vi "LV_beta.vi"() -> ()   [LabVIEW 2021]
uses:
  <vilib>/Analysis/NI_AALBase.lvlib
panel:
  out "Unscrambled":string
  out "Scrambled":string
  in  "Path 2":path
  out "Waveform Graph":dbl[](graph)
  out "length":i32
  in  "Path":path
  out "Display":string
  in  "CALC UI":T1
  in  "stop":bool
  out "Waveform Chart":dbl[](graph)
  out "String":string
  out "number (0 to 1)":dbl
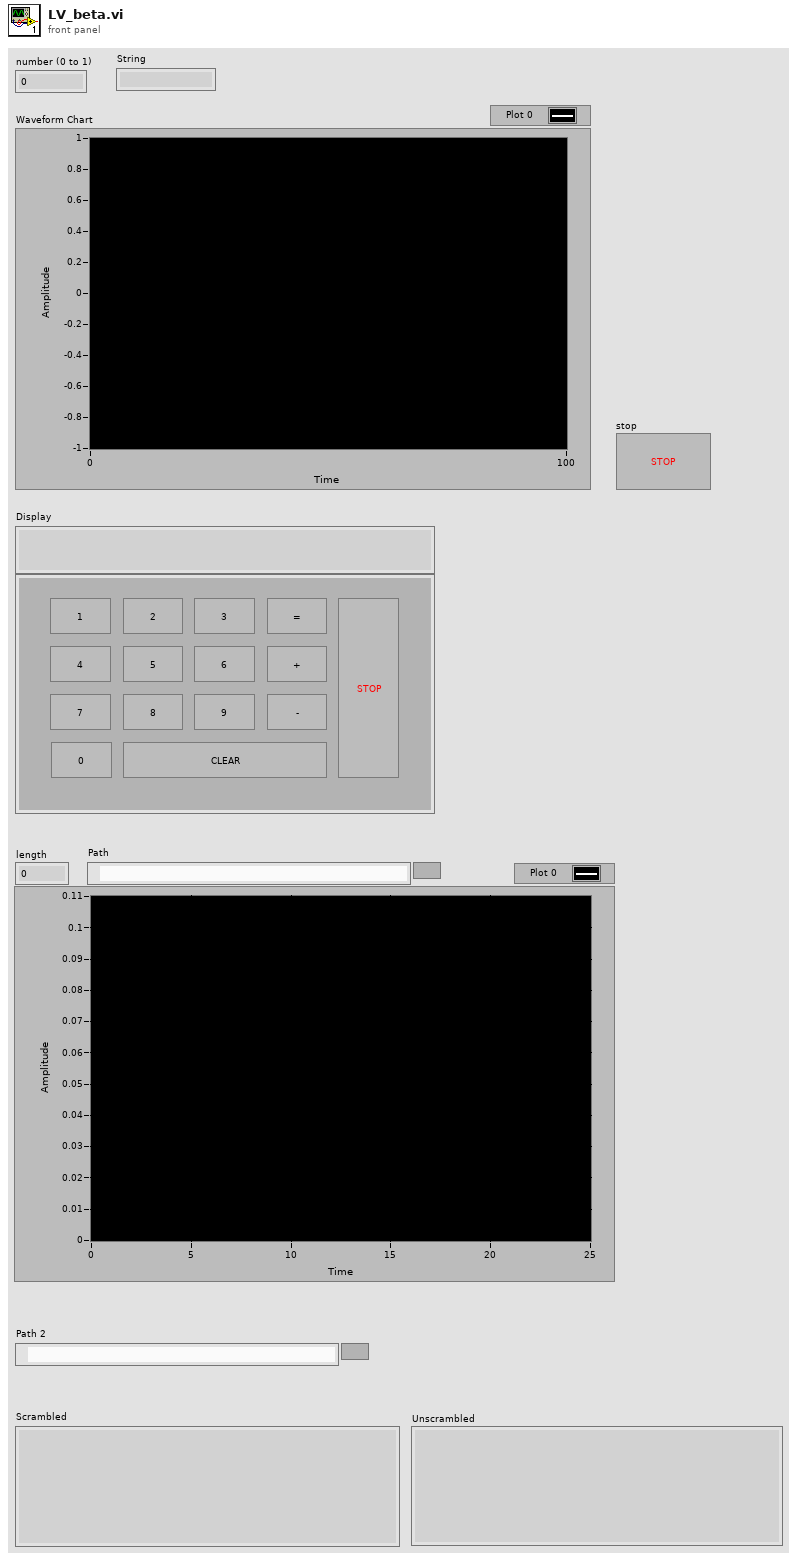
[diagram p1: front panel]
types:
  T1 = cluster{"1":bool, "2":bool, "3":bool, "Result":bool, "4":bool, "5":bool, "6":bool, "Add":bool, "7":bool, "8":bool, "9":bool, "Subtract":bool, "0":bool, "CLEAR":bool, "stop":bool}
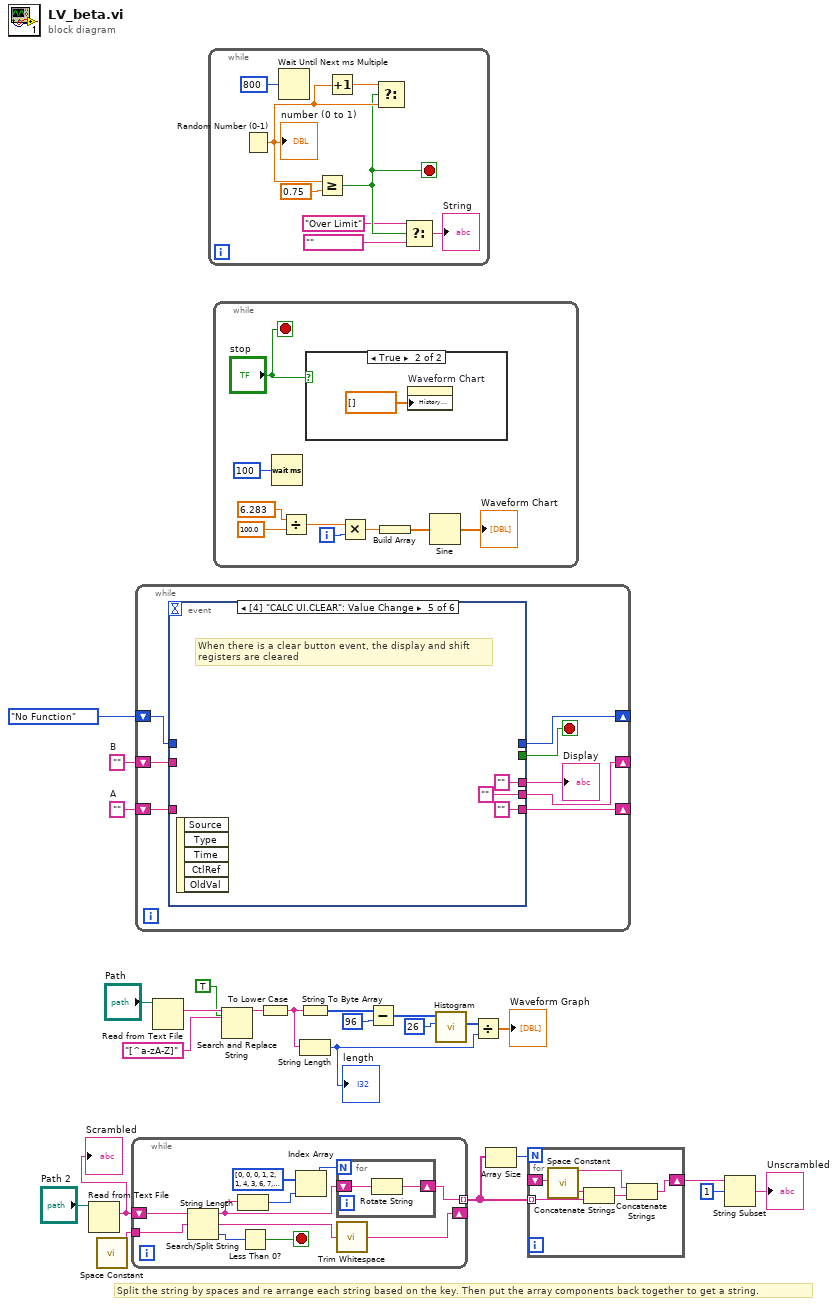
[diagram p0: block diagram]
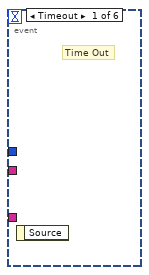
[diagram p2: hidden frame]
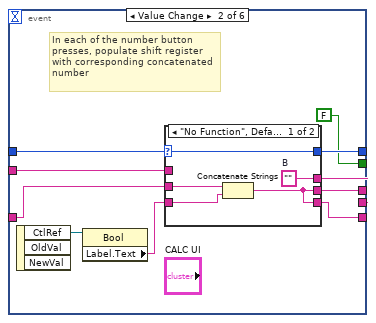
[diagram p3: hidden frame]
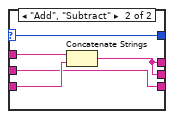
[diagram p4: hidden frame]
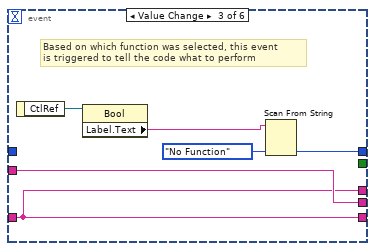
[diagram p5: hidden frame]
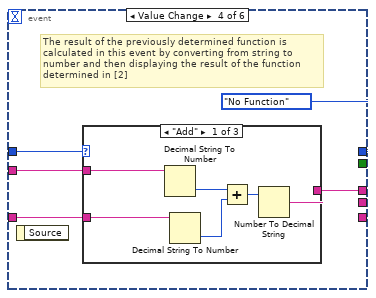
[diagram p6: hidden frame]
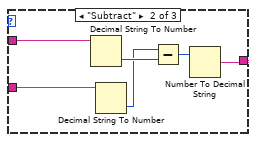
[diagram p7: hidden frame]
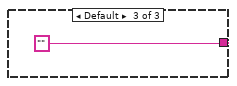
[diagram p8: hidden frame]
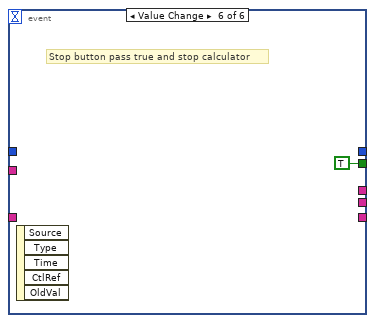
[diagram p9: hidden frame]
diagram:
  w19 = TRUE
  w23 = ""  # A
  w24 = ""  # B
  # "Split the string by spaces and re arrange each string based on the key. Then put the array components back together to get a string."
  n1 = Read from Text File(file (use dialog)="Path 2") -> (text=w7:string)  [unwired: 3 in, 3 out]
  "Scrambled" <- w7
  n2 = call <vilib>:"Space Constant.vi"() -> ("String"=w6:string)
  n3 = while {
    shift-right: [w33] -> _
    shift-left: w7 -> [w35]
    tunnel: [w25] -> w4 mode=indexing
    tunnel: w6 -> [w27]
    stop <- w31 stop-if-true
    n4 = Search/Split String(string=w35, search string/char (-)=w27) -> (substring before match=w26:string, match + rest of string=w34:string, offset of match=w32:i32)  [unwired: 1 in]
    n5 = String Length(string=w26) -> (length=w29:i32)
    n6 = Less Than 0?(x=w32) -> (x < 0?=w31:bool)
    n7 = Index Array(array=i32[] [0, 0, 0, 1, 2, 1, 4, 3, 6, 7, 6, 0, 0, 4], index=w29) -> (element=w28:i32)
    n8 = for {
      N: w28 -> [_]
      shift-right: [w36] -> w25
      shift-left: w26 -> [w37]
      n9 = Rotate String(1:w37) -> (0:w36:string)
    }
    n10 = call <vilib>:"Trim Whitespace.vi"("string"=w34) -> ("trimmed string"=w33:string)  [unwired: 1 in]
  }
  n11 = while {
    shift-right: [w41] -> _
    shift-left: w24 -> [w44]
    shift-right: [w40] -> _
    shift-left: w23 -> [w45]
    shift-right: [w42] -> _
    shift-left: enum16{"No Function", "Add", "Subtract"}."No Function" -> [w43]
    stop <- w39 stop-if-true
    n12 = event shown="[4] \"CALC UI.CLEAR\": Value Change" {
      selector: _ -> [_ _ _ _ _ _]
      dyn-events: _ -> [_ _ _ _ _ _]
      timeout: _ -> [_ _ _ _ _ _]
      tunnel: w45 -> [_ w53 w67 w73 _ _]
      tunnel: w44 -> [_ w47 w71 w74 _ _]
      tunnel: w43 -> [_ w54 _ w76 _ _]
      tunnel: [_ w51 w68 enum16{"No Function", "Add", "Subtract"}."No Function" _ _] -> w42
      tunnel: [_ w50 w71 _ "" ("B") _] -> w41
      tunnel: [_ w49 w67 _ "" ("A") _] -> w40
      tunnel: [_ FALSE _ _ _ TRUE] -> w39
      tunnel: [_ w46 w67 w72 "" ("A") _] -> w38
      event Timeout {
        # "Time Out"
        n13 = event-data() -> ()  [unwired: 1 in, 1 out]
      }
      event "CALC UI.1", "CALC UI.2", "CALC UI.3", "CALC UI.4", "CALC UI.5", "CALC UI.6", "CALC UI.7", "CALC UI.8", "CALC UI.9", "CALC UI.0": Value Change {
        # "In each of the number button presses, populate shift register with corresponding concatenated number"
        n14 = event-data() -> ("CtlRef"=w55:refnum<vi>)  [unwired: 1 in, 2 out]
        n15 = property class="Bool"(reference=w55) -> ("Label.Text"=w52:string)  [unwired: 1 in, 2 out]
        n16 = case shown="\"No Function\", Default" w54 {
          selector: w54 -> [w58 w62]
          tunnel: w53 -> [w60 w63]
          tunnel: w52 -> [w59 w64]
          tunnel: [w58 w62] -> w51
          tunnel: [w57 w61] -> w50
          tunnel: [w56 w63] -> w49
          tunnel: w47 -> [_ w65]
          tunnel: [w56 w61] -> w46
          frame "No Function", Default {
            w57 = ""  # B
            n17 = Concatenate Strings(w60, w59) -> (w56:string)
          }
          frame "Add", "Subtract" {
            n18 = Concatenate Strings(w65, w64) -> (w61:string)
          }
        }
      }
      event "CALC UI.Add", "CALC UI.Subtract": Value Change {
        # "Based on which function was selected, this event \nis triggered to tell the code what to perform"
        n19 = event-data() -> ("CtlRef"=w70:refnum<vi>)  [unwired: 1 in]
        n20 = property class="Bool"(reference=w70) -> ("Label.Text"=w66:string)  [unwired: 1 in, 2 out]
        n21 = Scan From String "Scan From String"(input string=w66, default 1=enum16{"No Function", "Add", "Subtract"}."No Function") -> (output 1=w68:enum16{"No Function", "Add", "Subtract"})  [unwired: 3 in, 3 out]
      }
      event "CALC UI.Result": Value Change {
        # "The result of the previously determined function is \ncalculated in this event by converting from string to \nnumber and then displaying the result of the function\ndetermined in [2]"
        n22 = event-data() -> ()  [unwired: 1 in, 1 out]
        n23 = case shown="\"Add\"" w76 {
          tunnel: w74 -> [w82 w88 _]
          tunnel: w73 -> [w81 w87 _]
          tunnel: [w77 w83 ""] -> w72
          frame "Add" {
            n24 = Decimal String To Number(string=w82) -> (number=w80:i32)  [unwired: 2 in, 1 out]
            n25 = Decimal String To Number(string=w81) -> (number=w79:i32)  [unwired: 2 in, 1 out]
            n26 = Add(x=w80, y=w79) -> (x+y=w78:i32)
            n27 = Number To Decimal String(number=w78) -> (decimal integer string=w77:string)  [unwired: 1 in]
          }
          frame "Subtract" {
            n28 = Decimal String To Number(string=w88) -> (number=w86:i32)  [unwired: 2 in, 1 out]
            n29 = Decimal String To Number(string=w87) -> (number=w85:i32)  [unwired: 2 in, 1 out]
            n30 = Subtract(x=w85, y=w86) -> (x-y=w84:i32)
            n31 = Number To Decimal String(number=w84) -> (decimal integer string=w83:string)  [unwired: 1 in]
          }
          frame Default {
          }
        }
      }
      event "CALC UI.CLEAR": Value Change {
        # "When there is a clear button event, the display and shift\nregisters are cleared"
        n32 = event-data() -> ()  [unwired: 1 in, 5 out]
      }
      event "CALC UI.stop": Value Change {
        # "Stop button pass true and stop calculator"
        n33 = event-data() -> ()  [unwired: 1 in, 5 out]
      }
    }
    "Display" <- w38
  }
  n34 = Read from Text File(file (use dialog)="Path") -> (text=w20:string)  [unwired: 3 in, 3 out]
  n35 = while {
    stop <- w98 stop-if-true
    n36 = Random Number (0-1)() -> (number: 0 to 1=w99:dbl)
    "number (0 to 1)" <- w99
    n37 = Wait Until Next ms Multiple(millisecond multiple=u32 800) -> ()  [unwired: 1 out]
    n38 = Greater Or Equal?(x=w99, y=0.75) -> (x >= y?=w98:bool)
    n39 = Increment(x=w99) -> (x+1=w100:dbl)
    n40 = Select(t=w100, s=w98, f=w99) -> ()  [unwired: 1 out]
    n41 = Select(t="Over Limit", s=w98, f="") -> (s? t:f=→"String":string)
  }
  n42 = while {
    i -> [w106]
    stop <- "stop" stop-if-true
    n43 = Wait (ms)(milliseconds to wait=u32 100) -> ()  [unwired: 1 out]
    n44 = Divide(x=6.283, y=100.0) -> (x/y=w107:dbl)
    n45 = case shown="True" "stop" {
      frame False {
      }
      frame True {
        n46 = property on="Waveform Chart" class="WFChart (strict)"("History Data"=dbl[] []) -> ()  [unwired: 2 in, 2 out]
      }
    }
    n47 = Multiply(x=w107, y=w106) -> (x*y=w105:dbl)
    n48 = Build Array(w105) -> (w104:dbl[])
    n49 = Sine(x=w104) -> (sin(x)=→"Waveform Chart":dbl[])
  }
  n50 = Search and Replace String(replace all?=w19, case sensitive?=w19, input string=w20, search string="[^a-zA-Z]") -> (result string=w18:string)  [unwired: 4 in, 3 out]
  n51 = To Lower Case(string=w18) -> (all lower case string=w17:string)
  n52 = String To Byte Array(string=w17) -> (unsigned byte array=w10:u8[])
  n53 = String Length(string=w17) -> (length=w13:i32)
  "length" <- w13
  n54 = Subtract(x=w10, y=96) -> (x-y=w15:i32[])
  n55 = call <vilib>:"Histogram.vi"("intervals"=26, "X"=w15) -> ("Histogram: h(x)"=w12:i32[])  [unwired: 6 in, 3 out]
  n56 = Divide(x=w12, y=w13) -> (x/y=→"Waveform Graph":dbl[])
  n57 = Array Size(array=w4) -> (size(s)=w5:i32)
  n58 = for {
    N: w5 -> [_]
    shift-right: [w114] -> w2
    shift-left: _ -> [w113]
    tunnel: w4 -> [w116] mode=indexing
    n59 = call <vilib>:"Space Constant.vi"() -> ("String"=w112:string)
    n60 = Concatenate Strings(w112, w116) -> (w115:string)
    n61 = Concatenate Strings(w113, w115) -> (w114:string)
  }
  n62 = String Subset(string=w2, offset (0)=1) -> (substring=→"Unscrambled":string)  [unwired: 1 in]
